vi "image_reg_coke_can.vi"() -> ()   [LabVIEW 2012]
uses:
  Labmembers/Lukas Gemar/Control 1.ctl
  <vilib>/DAQmx/write.llb/DAQmx Write (Digital Bool 1Line 1Point).vi
  <vilib>/Analysis/baseanly.llb/Mean (DBL).vi
  <vilib>/DAQmx/create/channels.llb/DAQmx Create Channel (DO-Digital Output).vi
  <vilib>/DAQmx/miscellaneous.llb/DAQmx Fill In Error Info.vi
  <vilib>/Analysis/NI_AALBase.lvlib
panel:
  in  "Bin (n x n) 2":u16(ring)=1 caption="Cursor Bin" items=["1x1"=1, "2x2"=2, "4x4"=4]
  out "Status":string="Ready"
  in  "Tab Control":enum32{"Page 1", "Page 2", "Page 3"}(tab)
  out "Initialize":u32
  out "Initialize?":bool
  out "Bits per Channel":i32
  out "camera initialization error":errorcluster
  out "Camera ID":string="0"
  out "Model":string="0"
  out "y pixels":i32
  out "x pixels":i32
  out "Elapsed time (sec)":dbl=100.0 min=1.0 max=5000.0 step=1.0
  out "Total time (sec)":dbl=100.0 min=1.0 max=5000.0 step=1.0
  in  "# frames":u32=100
  in  "Acquire movie":bool
  in  "Previous ROI 2":bool
  out "Previous ROI":T1={"x offset"=256, "y offset"=256, "x width"=512, "y width"=512} caption="Previous" {"x offset" min=1 max=512 step=1; "y offset" min=1 max=512 step=1; "x width" min=1 max=512 step=1; "y width" min=1 max=512 step=1}
  in  "Update ROI":bool
  out "ROI":T1={"x offset"=960, "y offset"=912, "x width"=136, "y width"=152} caption="Current" {"x offset" min=1 max=512 step=1; "y offset" min=1 max=512 step=1; "x width" min=1 max=512 step=1; "y width" min=1 max=512 step=1}
  in  "Bin (n x n)":u16(ring)=1 caption="Cursor Bin" items=["1x1"=1, "2x2"=2, "4x4"=4]
  in  "Symmetrical":bool=TRUE
  in  "Define ROI":bool
  in  "ROI selection":u16(ring)=2 items=["Full ROI", "Central quad", "Custom ROI"]
  out "Frames Recorded":i32
  in  "Movie name":string
  in  "Register!":bool
  in  "Image Registration":bool
  in  "Stop Program":bool
  in  "Enter Live Mode":bool
  out "Image":i32[][](graph)
  out "mean":dbl=701.2764784557547
  out "max value":u16=1056
  out "min value":u16=384
  out "Histogram":T2(graph)={"X Values"=[417.6, 484.8, 552.0, 619.2, 686.4, 753.6, 820.8, 888.0, 955.2, 1022.4], "Histogram: h(x)"=[403, 4234, 6440, 8496, 9541, 10568, 10361, 4568, 669, 48]}
  out "Camera Error":errorcluster
  in  "base path":path=path "C:/Peng/Data"
  in  "Exposure (msec)":T3=100.0
  out "Location indicator":u16[][](graph)
  out "max frame rate (Hz)":dbl
  in  "Image Reg Path":path=path "C:/data/Lukas_data/image_reg.bin"
  out "DeviceID":u32
  out "SequID":u32
  in  "DMD_trigger":tag="Dev1/port0/line0" caption="DMD trigger"
  in  "DAQ Error":errorcluster
  in  "Image Reg ctl points":path=path "C:/data/Lukas_data/image_reg.txt"
  in  "Transformation":path=path "C:/data/Lukas_data/transform.txt"
  out "DevFreeErr":i32
  out "SeqFreeErr":i32
  out "ALP_Error":errorcluster
  out "Previous Bin":u16(ring)=2 caption="Cursor Bin" items=["1x1"=1, "2x2"=2, "4x4"=4]
  out "ROI cursor":T1={"x offset"=480, "y offset"=456, "x width"=68, "y width"=76} {"x offset" min=1 max=512 step=1; "y offset" min=1 max=512 step=1; "x width" min=1 max=512 step=1; "y width" min=1 max=512 step=1}
  # "ROI control"
  # "Focus mode settings"
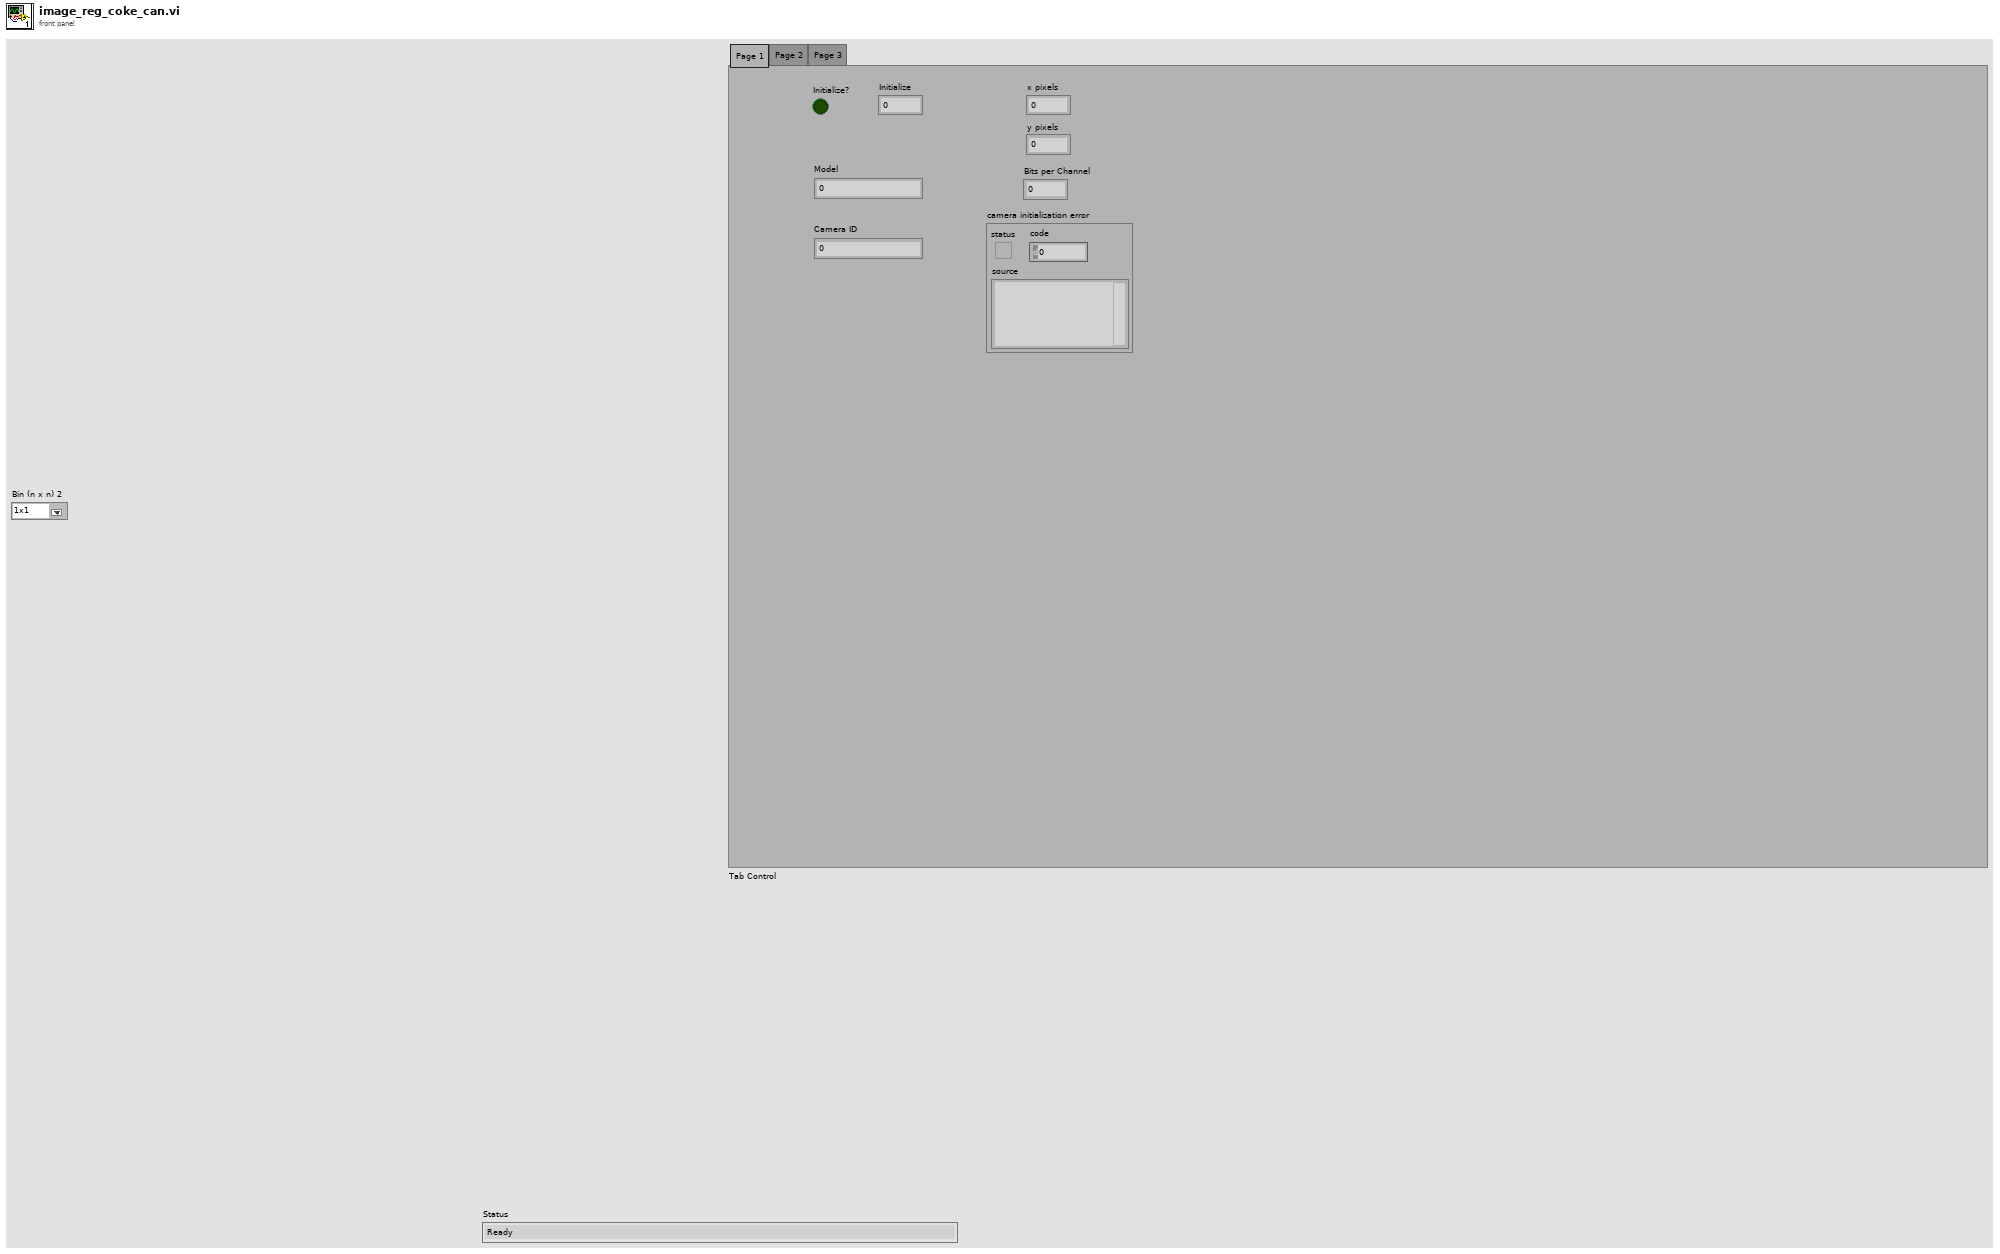
[diagram p1: front panel]
types:
  T1 = cluster{"x offset":i32, "y offset":i32, "x width":i32, "y width":i32}
  T2 = cluster{"X Values":dbl[], "Histogram: h(x)":i32[]}
  T3 = typedef "Control 1.ctl" = dbl
  T4 = cluster{"width":u32, "height":u32, "datatype":u32}
  T5 = enum8{"Enabled", "Disabled", "Disabled and Grayed Out"}
  T6 = cluster{"Horizontal Offset":i32, "Vertical Offset":i32, "Horizontal Width":i32, "Vertical Width":i32}
  T7 = cluster{"Value":i32, "Minimum":i32, "Maximum":i32, "Increment":i32}
  T8 = cluster{"X min":dbl, "Y min":dbl, "X max":dbl, "Y max":dbl}
  T9 = cluster{"Cursor.Cursor X":dbl, "Cursor.Cursor Y":dbl, "Cursor.Cursor X":dbl, "Cursor.Cursor Y":dbl}
  T10 = cluster{"Cursor1. X":dbl, "Cursor1. Y":dbl, "Cursor2. X":dbl, "Cursor2. Y":dbl}
  T11 = cluster{"x offset":dbl, "y offset":dbl, "x width":dbl, "y width":dbl}
  T12 = typedef "LVPointDoubleTypeDef.ctl" = cluster{"Cursor X":dbl, "Cursor Y":dbl}
  T13 = cluster{"XScale.Minimum":dbl, "YScale.Minimum":dbl, "XScale.Maximum":dbl, "YScale.Maximum":dbl}
  T14 = cluster{"Cursor.Cursor Position":T12, "Cursor.Cursor Position":T12}
  T15 = cluster{"Cursor1.Position":T12, "Cursor2.Position":T12}
  T16 = cluster{"Active Cursor":u32, "Active Cursor":u32, dbl, dbl}
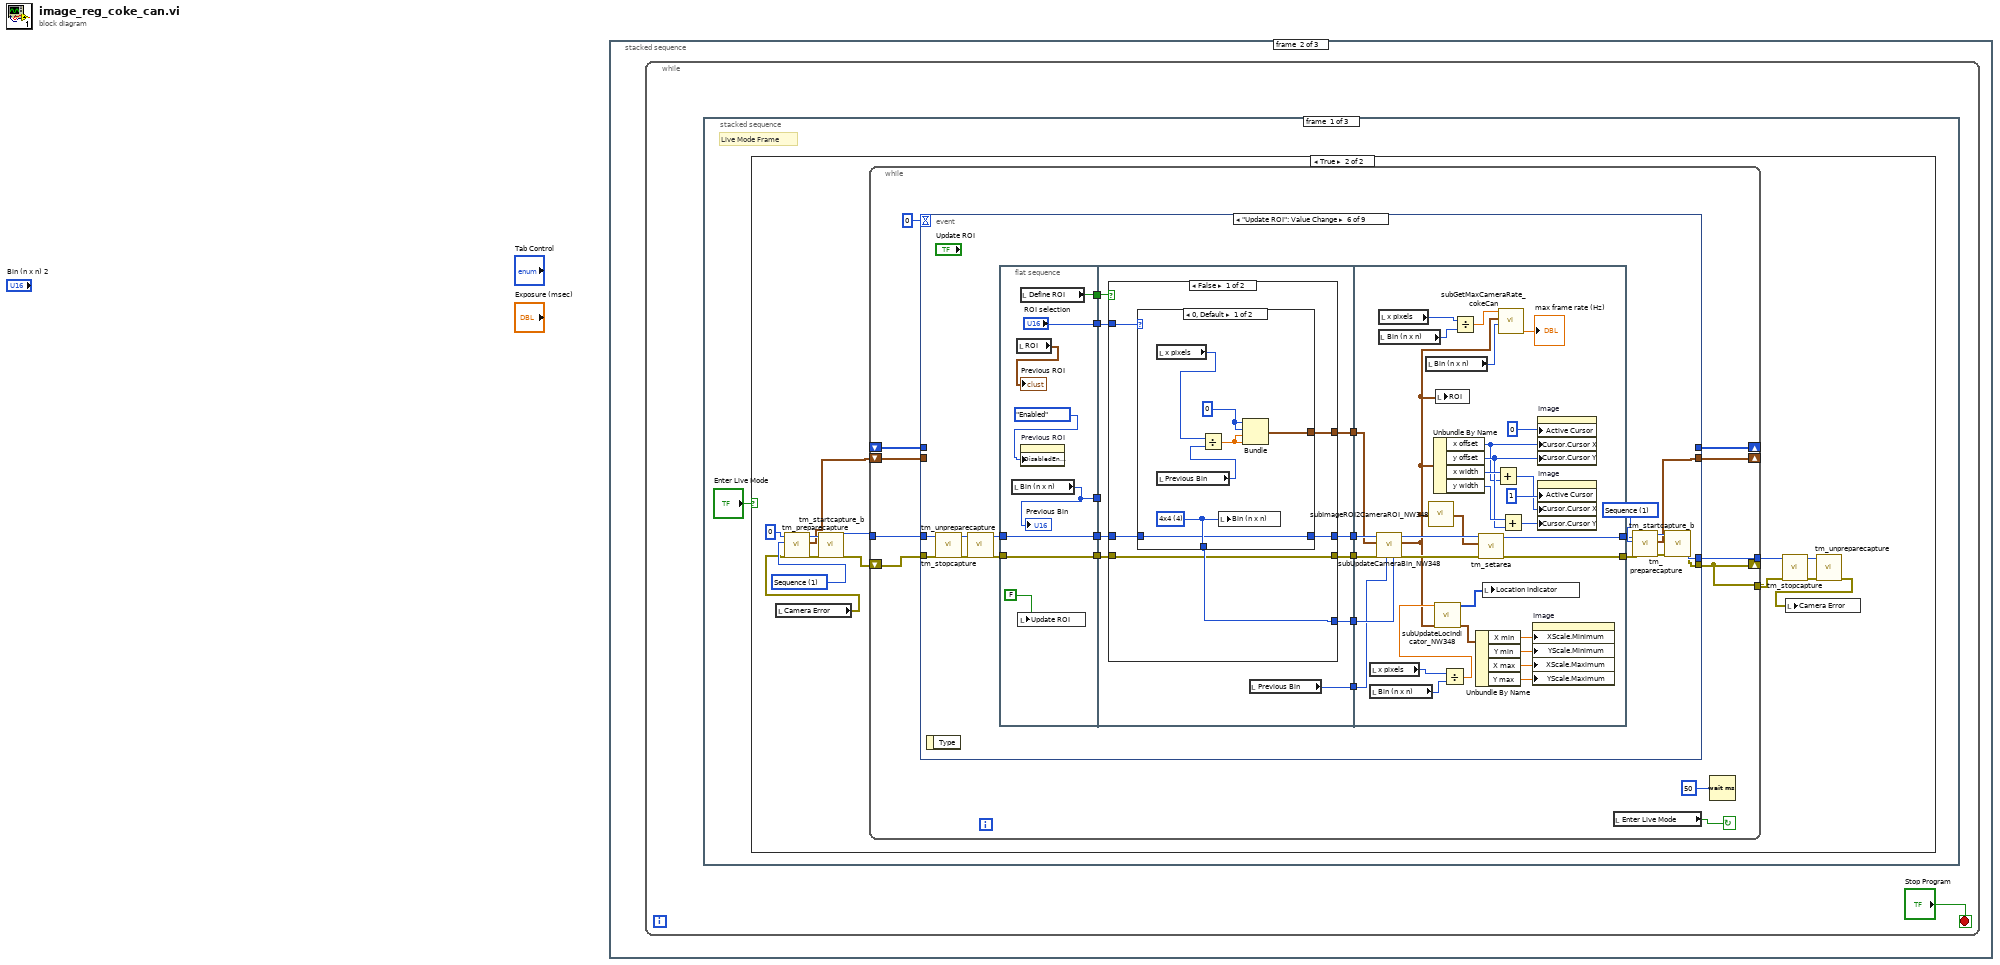
[diagram p0: block diagram]
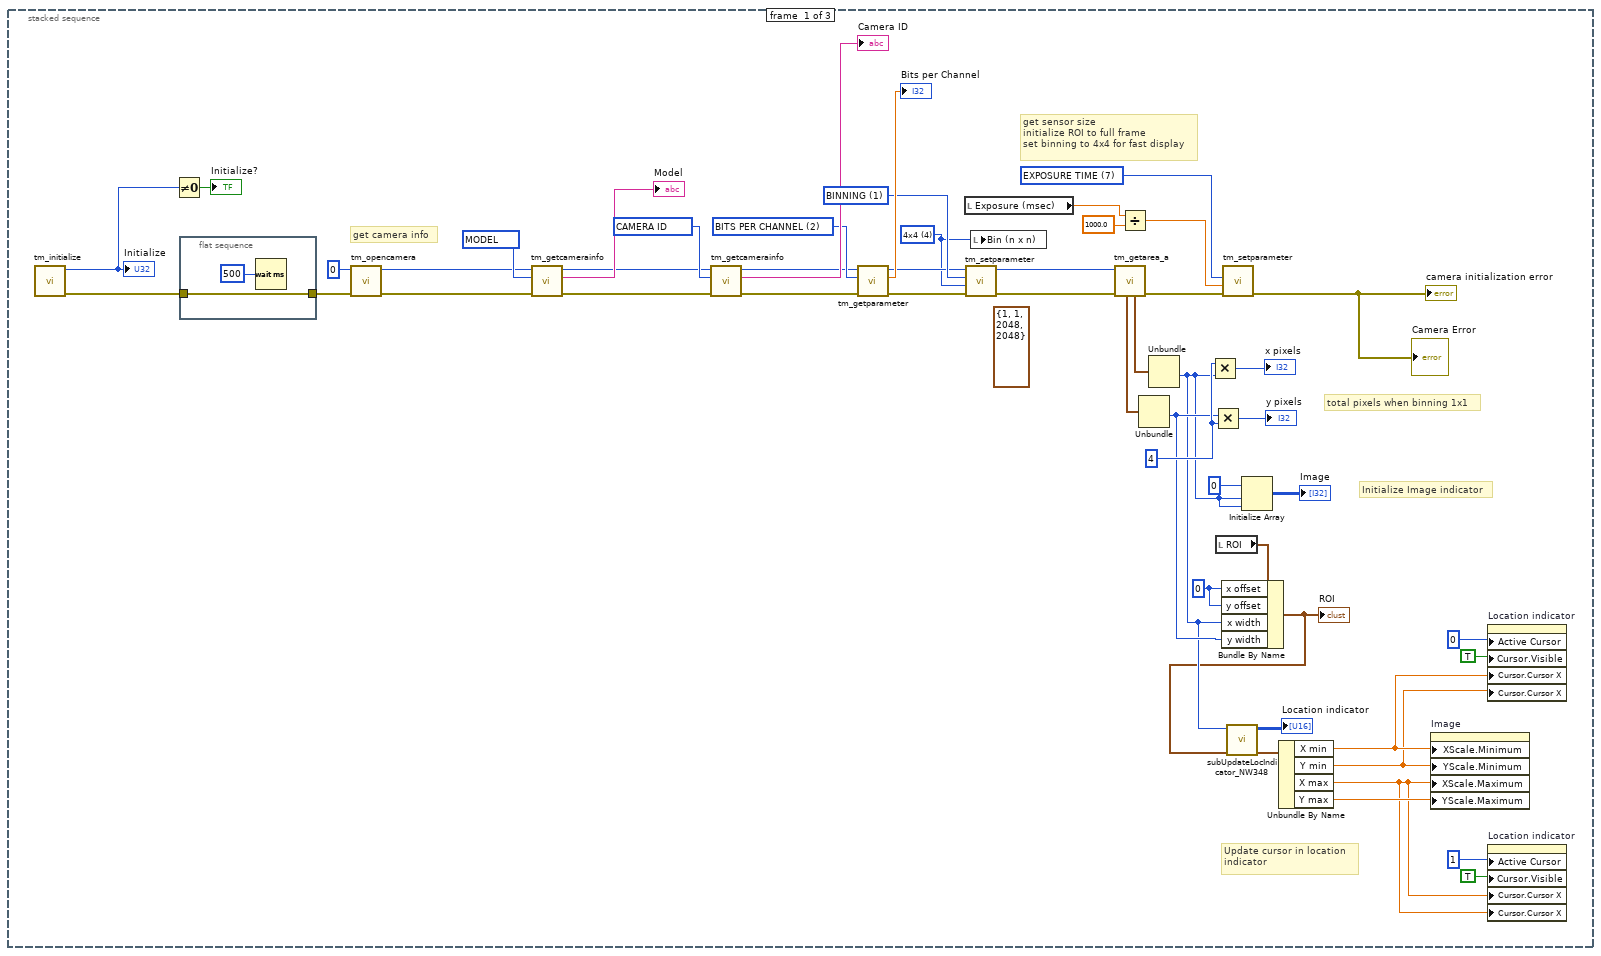
[diagram p2: hidden frame]
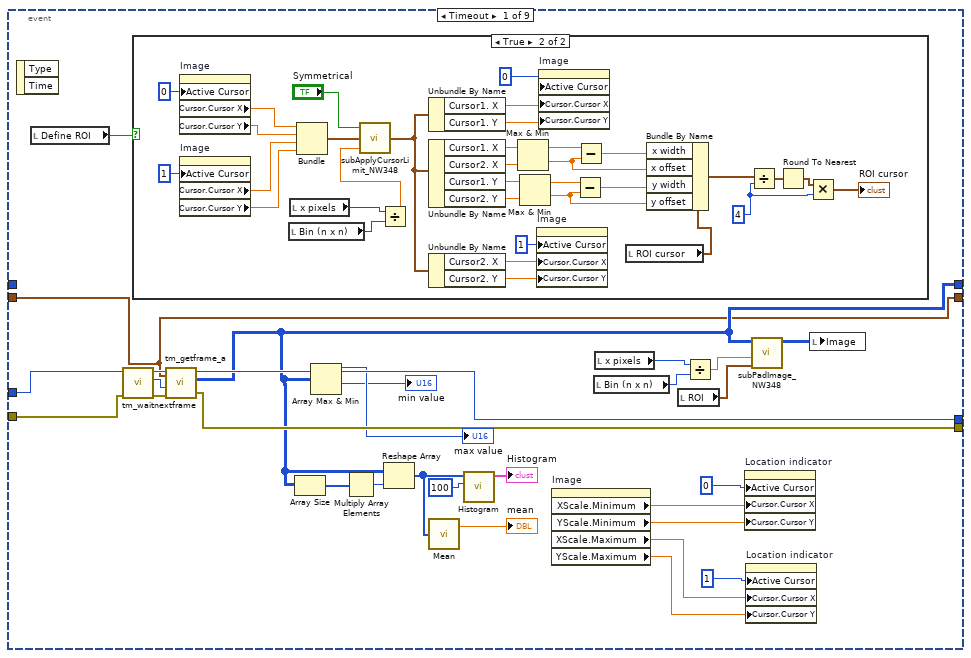
[diagram p4: hidden frame]
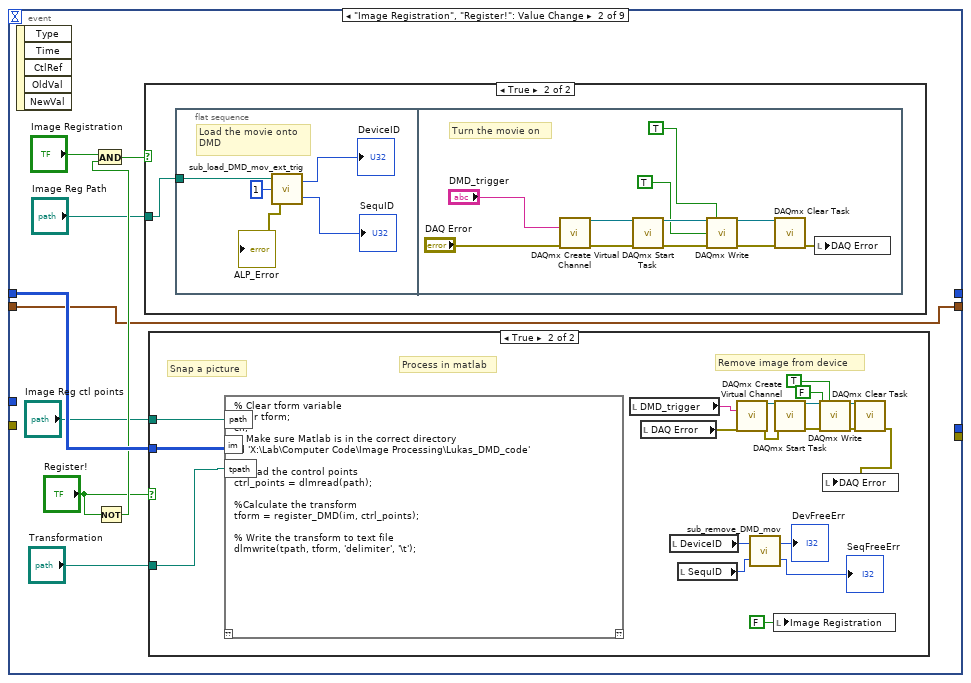
[diagram p6: hidden frame]
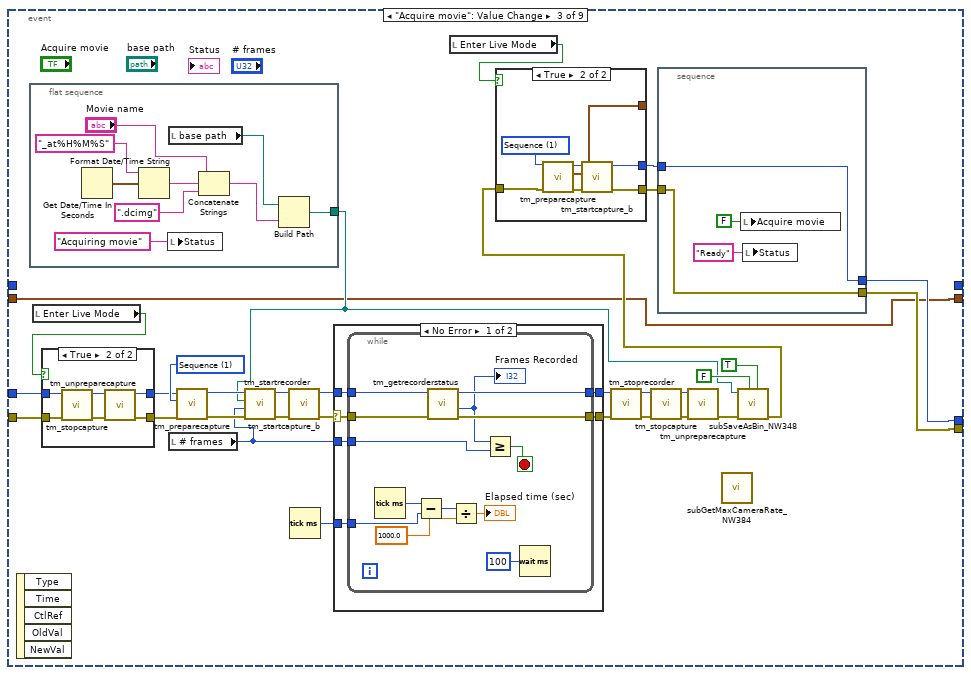
[diagram p9: hidden frame]
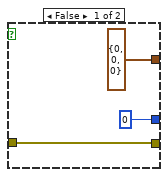
[diagram p10: hidden frame]
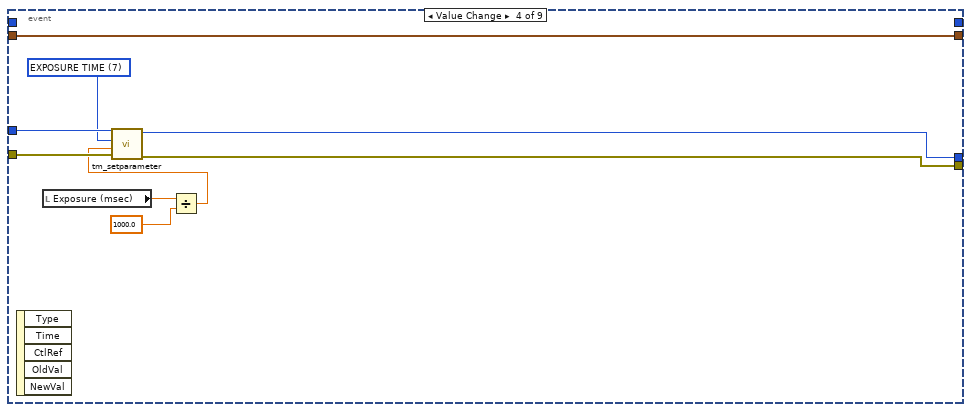
[diagram p13: hidden frame]
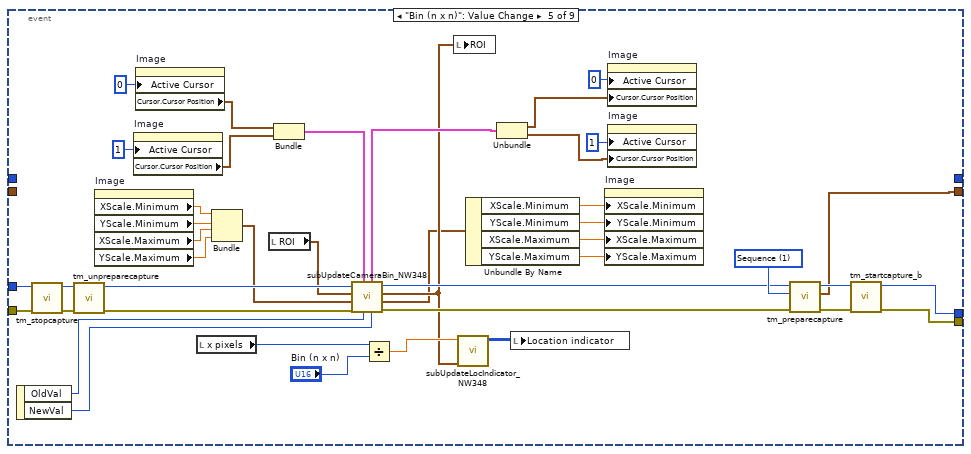
[diagram p14: hidden frame]
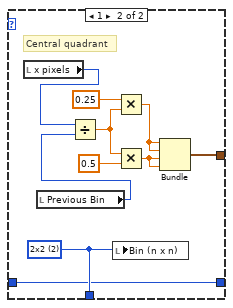
[diagram p15: hidden frame]
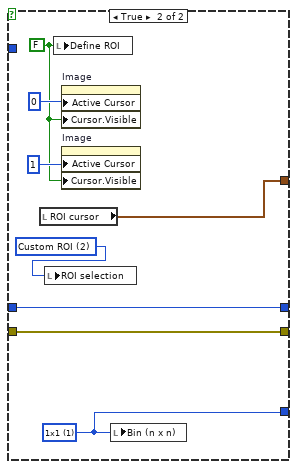
[diagram p16: hidden frame]
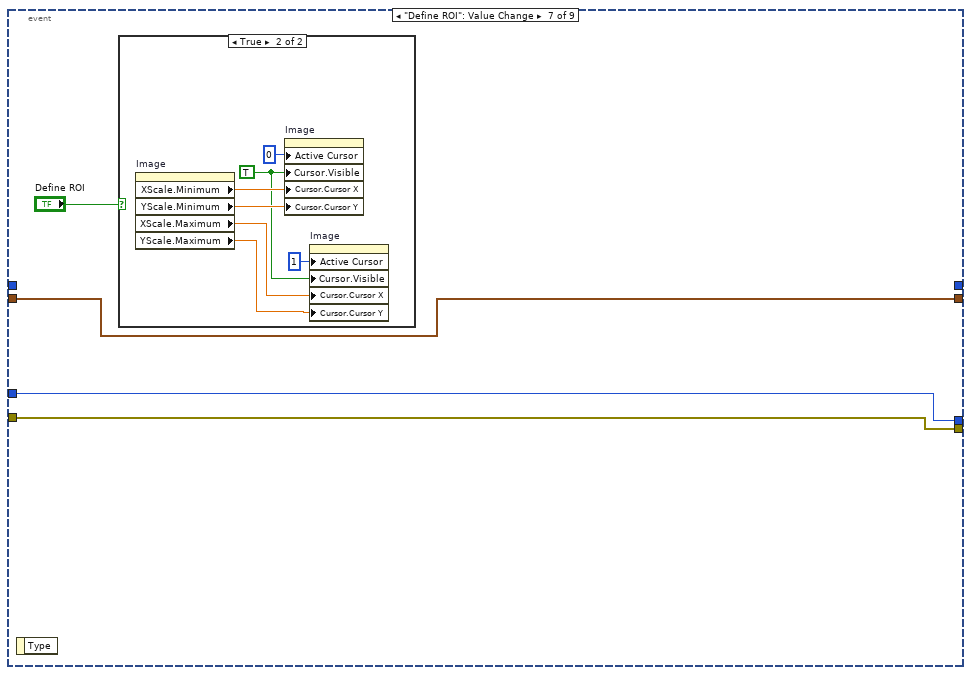
[diagram p17: hidden frame]
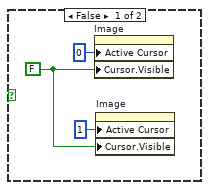
[diagram p18: hidden frame]
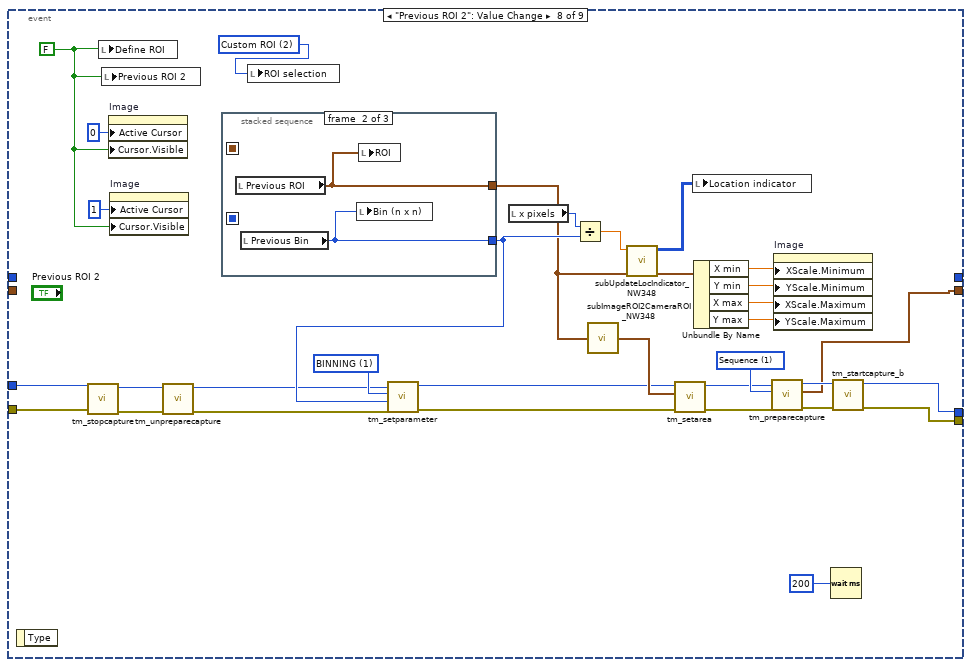
[diagram p19: hidden frame]
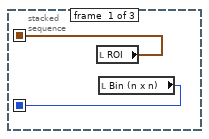
[diagram p20: hidden frame]
diagram:
  n1 = stacked-sequence {
    frame #0 {
      w16 = 0 ("x offset")
      w28 = 4
      (unwired) T6 {"Horizontal Offset"=1, "Vertical Offset"=1, "Horizontal Width"=2048, "Vertical Width"=2048} ("Sub Region")
      w1 = u16 4 items=["1x1"=1, "2x2"=2, "4x4"=4] ("Bin (n x n)")
      w35 = 7 items=["BINNING"=1, "BITS PER CHANNEL"=2, "ACTIVE VIEW INDEX"=3, "CCD MODE"=4, "SENSOR MODE"=5, "READOUT MODE"=6, "EXPOSURE TIME"=7, "CONTRAST GAIN"=8, "CONTRAST OFFSET"=9, "LIGHT MODE"=10, "SENSITIVITY"=11, "WHITE BALANCE"=12, "PHOTON IMAGING MODE"=13, "HIGH DYNAMIC RANGE MODE"=14, "TRIGGER SOURCE"=15, "TRIGGER ACTIVE"=16, "TRIGGER MODE"=17, "TRIGGER POLARITY"=18, "TRIGGER GLOBAL EXPOSURE"=19, "FIRST TRIGGER BEHAVIOR"=20, "TRIGGER TIMES"=21, "OUTPUT TRIGGER POLARITY"=22, "OUTPUT TRIGGER DELAY"=23, "OUTPUT TRIGGER PERIOD"=24, "TEMPERATURE"=25, "TEMPERATURE TARGET"=26, "SENSOR COOLER FAN"=27, "MECHANICAL SHUTTER"=28, "BACK FOCUS POSITION"=29, "FRAMEBUNDLE MODE"=30, "FRAMEBUNDLE NUMBER"=31, "LINEBUNDLE HEIGHT"=32, "TRIGGER CONNECTOR"=33, "IMAGE PIXEL TYPE"=34] ("Parameter")
      w39 = 1 items=["BINNING"=1, "BITS PER CHANNEL"=2, "ACTIVE VIEW INDEX"=3, "CCD MODE"=4, "SENSOR MODE"=5, "READOUT MODE"=6, "EXPOSURE TIME"=7, "CONTRAST GAIN"=8, "CONTRAST OFFSET"=9, "LIGHT MODE"=10, "SENSITIVITY"=11, "WHITE BALANCE"=12, "PHOTON IMAGING MODE"=13, "HIGH DYNAMIC RANGE MODE"=14, "TRIGGER SOURCE"=15, "TRIGGER ACTIVE"=16, "TRIGGER MODE"=17, "TRIGGER POLARITY"=18, "TRIGGER GLOBAL EXPOSURE"=19, "FIRST TRIGGER BEHAVIOR"=20, "TRIGGER TIMES"=21, "OUTPUT TRIGGER POLARITY"=22, "OUTPUT TRIGGER DELAY"=23, "OUTPUT TRIGGER PERIOD"=24, "TEMPERATURE"=25, "TEMPERATURE TARGET"=26, "SENSOR COOLER FAN"=27, "MECHANICAL SHUTTER"=28, "BACK FOCUS POSITION"=29, "FRAMEBUNDLE MODE"=30, "FRAMEBUNDLE NUMBER"=31, "LINEBUNDLE HEIGHT"=32, "TRIGGER CONNECTOR"=33, "IMAGE PIXEL TYPE"=34] ("Parameter")
      w41 = 2 items=["BINNING"=1, "BITS PER CHANNEL"=2, "ACTIVE VIEW INDEX"=3, "CCD MODE"=4, "SENSOR MODE"=5, "READOUT MODE"=6, "EXPOSURE TIME"=7, "CONTRAST GAIN"=8, "CONTRAST OFFSET"=9, "LIGHT MODE"=10, "SENSITIVITY"=11, "WHITE BALANCE"=12, "PHOTON IMAGING MODE"=13, "HIGH DYNAMIC RANGE MODE"=14, "TRIGGER SOURCE"=15, "TRIGGER ACTIVE"=16, "TRIGGER MODE"=17, "TRIGGER POLARITY"=18, "TRIGGER GLOBAL EXPOSURE"=19, "FIRST TRIGGER BEHAVIOR"=20, "TRIGGER TIMES"=21, "OUTPUT TRIGGER POLARITY"=22, "OUTPUT TRIGGER DELAY"=23, "OUTPUT TRIGGER PERIOD"=24, "TEMPERATURE"=25, "TEMPERATURE TARGET"=26, "SENSOR COOLER FAN"=27, "MECHANICAL SHUTTER"=28, "BACK FOCUS POSITION"=29, "FRAMEBUNDLE MODE"=30, "FRAMEBUNDLE NUMBER"=31, "LINEBUNDLE HEIGHT"=32, "TRIGGER CONNECTOR"=33, "IMAGE PIXEL TYPE"=34] ("Parameter")
      w45 = u32 67109122 items=["BUS"=67109121, "CAMERA ID"=67109122, "VENDOR"=67109123, "MODEL"=67109124, "CAMERA VERSION"=67109125, "DRIVER VERSION"=67109126, "MODULE VERSIOIN"=67109127, "DCAMAPI VERSION"=67109128] ("Info ID")
      w44 = u32 67109124 items=["BUS"=67109121, "CAMERA ID"=67109122, "VENDOR"=67109123, "MODEL"=67109124, "CAMERA VERSION"=67109125, "DRIVER VERSION"=67109126, "MODULE VERSIOIN"=67109127, "DCAMAPI VERSION"=67109128] ("Info ID")
      # "Update cursor in location\nindicator"
      # "total pixels when binning 1x1"
      # "Initialize Image indicator"
      # "get sensor size\ninitialize ROI to full frame\nset binning to 4x4 for fast display"
      # "get camera info"
      n2 = call <userlib>:"tm_initialize.vi"() -> ("error out"=w38:errorcluster, "Number Of Cameras"=w49:u32)  [unwired: 10 in]
      "Initialize" <- w49
      n3 = Not Equal To 0?(x=w49) -> (x != 0?=→"Initialize?":bool)
      n4 = flat-sequence {
        tunnel: w38 -> [w52]
        tunnel: [w52] -> w37
        frame #0 {
          n5 = Wait (ms)(milliseconds to wait=u32 500) -> ()  [unwired: 1 out]
        }
      }
      n6 = call <userlib>:"tm_opencamera.vi"("error in (no error)"=w37, "Camera Index"=u32 0 ("milliseconds to wait")) -> ("error out"=w47:errorcluster, "Handle out"=w25:u32)  [unwired: 8 in]
      n7 = call <userlib>:"tm_getcamerainfo.vi"("error in (no error)"=w47, "Info ID"=w44, "Handle in"=w25) -> ("error out"=w43:errorcluster, "String"=→"Model":string, "Handle out"=w24:u32)  [unwired: 6 in]
      n8 = call <userlib>:"tm_getcamerainfo.vi"("error in (no error)"=w43, "Info ID"=w45, "Handle in"=w24) -> ("error out"=w32:errorcluster, "String"=→"Camera ID":string, "Handle out"=w23:u32)  [unwired: 6 in]
      n9 = call <userlib>:"tm_getparameter.vi"("error in (no error)"=w32, "Parameter"=w41, "Handle in"=w23) -> ("error out"=w34:errorcluster, "Value out"=→"Bits per Channel":dbl, "Handle out"=w22:u32)  [unwired: 6 in]
      n10 = local read "Exposure (msec)"() -> (w21:T3)
      n11 = call <userlib>:"tm_setparameter.vi"("error in (no error)"=w34, "Value in"=w1, "Parameter"=w39, "Handle in"=w22) -> ("error out"=w9:errorcluster, "Handle out"=w10:u32)  [unwired: 6 in]
      n12 = local write "Bin (n x n)"(w1) -> ()
      n13 = call <userlib>:"tm_getarea_a.vi"("error in (no error)"=w9, "Handle in"=w10) -> ("error out"=w36:errorcluster, "H Width"=w30:T7, "V Width"=w29:T7)  [unwired: 4 in, 3 out]
      n14 = Divide(x=w21, y=1000.0) -> (x/y=w50:T3)
      n15 = Unbundle(w29) -> ("Maximum"=w17:i32)  [unwired: 3 out]
      n16 = Unbundle(w30) -> ("Maximum"=w15:i32)  [unwired: 3 out]
      n17 = Multiply(x=w28, y=w15) -> (x*y=→"x pixels":i32)
      n18 = Multiply(x=w17, y=w28) -> (x*y=→"y pixels":i32)
      n19 = local read "ROI"() -> (w18:T1)
      n20 = Bundle By Name(cluster=w18, "x offset"=w16, "y offset"=w16, "x width"=w15, "y width"=w17) -> (w14:T1)
      "ROI" <- w14
      n21 = call <userlib>:"tm_setparameter.vi"("error in (no error)"=w36, "Value in"=w50, "Parameter"=w35) -> ("error out"=→"camera initialization error" →"Camera Error":errorcluster)  [unwired: 7 in, 1 out]
      n22 = call "subUpdateLocIndicator_NW348.vi"("ROI"=w14, "pixel range"=w15) -> ("Graph scale"=w13:T8, "Location indicator"=→"Location indicator":u16[][])  [unwired: 8 in]
      n23 = Initialize Array(0, w15, w15) -> (→"Image":i32[][])
      n24 = Unbundle By Name(w13) -> ("X min"=w6:dbl, "Y min"=w5:dbl, "X max"=w2:dbl, "Y max"=w12:dbl)
      n25 = property on="Image" class="IntGraph (strict)"("XScale.Minimum"=w6, "YScale.Minimum"=w5, "XScale.Maximum"=w2, "YScale.Maximum"=w12) -> ()  [unwired: 2 in, 2 out]
      n26 = property on="Location indicator" class="IntGraph (strict)"("Active Cursor"=0 ("x offset"), "Cursor.Visible"=TRUE, "Cursor.Cursor X"=w6, "Cursor.Cursor X"=w5) -> ()  [unwired: 2 in, 2 out]
      n27 = property on="Location indicator" class="IntGraph (strict)"("Active Cursor"=1 ("x offset"), "Cursor.Visible"=TRUE, "Cursor.Cursor X"=w2, "Cursor.Cursor X"=w2) -> ()  [unwired: 2 in, 2 out]
    }
    frame #1 {
      n28 = while {
        stop <- "Stop Program" stop-if-true
        n29 = stacked-sequence {
          frame #0 {
            # "Live Mode Frame"
            n30 = case shown="True" "Enter Live Mode" {
              frame False {
              }
              frame True {
                w68 = 1 items=["Snap", "Sequence"] ("Capture mode")
                n31 = local read "Camera Error"() -> (w57:errorcluster)
                n32 = call <userlib>:"tm_preparecapture.vi"("error in (no error)"=w57, "Capture mode"=w68, "Handle in"=u32 0) -> ("error out"=w66:errorcluster, "Buffer"=w56:T4, "Handle out"=w67:u32)  [unwired: 5 in, 1 out]
                n33 = call <userlib>:"tm_startcapture_b.vi"("error in (no error)"=w66, "Handle in"=w67) -> ("error out"=w64:errorcluster, "Handle out"=w63:u32)  [unwired: 8 in]
                n34 = while {
                  tunnel: [w78] -> w59
                  shift-right: [w75] -> _
                  shift-left: w64 -> [w77]
                  tunnel: w63 -> [w76]
                  tunnel: [w75] -> w60
                  shift-right: [w72] -> _
                  shift-left: _ -> [w71]
                  shift-right: [w70] -> _
                  shift-left: w56 -> [w69]
                  stop <- w79 continue-if-true
                  n35 = event shown="[5] \"Update ROI\": Value Change" {
                    selector: _ -> [_ _ _ _ _ _ _ _ _]
                    dyn-events: _ -> [_ _ _ _ _ _ _ _ _]
                    timeout: 0 -> [_ _ _ _ _ _ _ _ _]
                    tunnel: [w108 _ w191 w277 w289 w335 w429 w450 _] -> w78
                    tunnel: w77 -> [w107 _ w218 w275 w320 w327 w428 w443 _]
                    tunnel: w76 -> [w106 _ w217 w279 w321 w326 w429 w444 _]
                    tunnel: [w105 _ w190 w276 w288 w334 w428 w449 _] -> w75
                    tunnel: [w81 _ _ _ _ _ _ _ _] -> w72
                    tunnel: w71 -> [_ w151 _ _ _ _ _ _ _]
                    tunnel: [w80 w143 w188 w271 w292 w333 w427 w442 w480] -> w70
                    tunnel: w69 -> [w80 w143 w188 w271 _ _ w427 _ w480]
                    event Timeout {
                      n36 = event-data() -> ()  [unwired: 1 in, 2 out]
                      n37 = local read "Define ROI"() -> (w95:bool)
                      n38 = call <userlib>:"tm_waitnextframe.vi"("error in (no error)"=w107, "Handle in"=w106) -> ("error out"=w97:errorcluster, "Frame Index"=w99:i32, "Handle out"=w98:u32)  [unwired: 6 in, 1 out]
                      n39 = case shown="True" w95 {
                        frame False {
                        }
                        frame True {
                          w110 = u32 4 ("Active Cursor")
                          n40 = property on="Image" class="IntGraph (strict)"("Active Cursor"=u32 0) -> ("Cursor.Cursor X"=w138:dbl, "Cursor.Cursor Y"=w137:dbl)  [unwired: 2 in, 2 out]
                          n41 = property on="Image" class="IntGraph (strict)"("Active Cursor"=u32 1) -> ("Cursor.Cursor X"=w140:dbl, "Cursor.Cursor Y"=w139:dbl)  [unwired: 2 in, 2 out]
                          n42 = local read "Bin (n x n)"() -> (w134:u16)
                          n43 = local read "x pixels"() -> (w133:i32)
                          n44 = Bundle("Cursor.Cursor X"=w138, "Cursor.Cursor Y"=w137, "Cursor.Cursor X"=w140, "Cursor.Cursor Y"=w139) -> (w136:T9)  [unwired: 1 in]
                          n45 = Divide(x=w133, y=w134) -> (x/y=w132:dbl)
                          n46 = call "subApplyCursorLimit_NW348.vi"("Cursor limit"=w132, "Cursor input"=w136, "Symmetrical ROI"="Symmetrical") -> ("Cursor output"=w131:T10)  [unwired: 2 in]
                          n47 = Unbundle By Name(w131) -> ("Cursor1. X"=w129:dbl, "Cursor1. Y"=w128:dbl)
                          n48 = Unbundle By Name(w131) -> ("Cursor1. X"=w124:dbl, "Cursor2. X"=w123:dbl, "Cursor1. Y"=w121:dbl, "Cursor2. Y"=w122:dbl)
                          n49 = Unbundle By Name(w131) -> ("Cursor2. X"=w126:dbl, "Cursor2. Y"=w125:dbl)
                          n50 = Max & Min(x=w124, y=w123) -> (max(x,y)=w120:dbl, min(x,y)=w118:dbl)
                          n51 = Max & Min(x=w121, y=w122) -> (max(x,y)=w119:dbl, min(x,y)=w115:dbl)
                          n52 = property on="Image" class="IntGraph (strict)"("Active Cursor"=u32 1, "Cursor.Cursor X"=w126, "Cursor.Cursor Y"=w125) -> ()  [unwired: 2 in, 2 out]
                          n53 = property on="Image" class="IntGraph (strict)"("Active Cursor"=u32 0, "Cursor.Cursor X"=w129, "Cursor.Cursor Y"=w128) -> ()  [unwired: 2 in, 2 out]
                          n54 = Subtract(x=w119, y=w115) -> (x-y=w116:dbl)
                          n55 = Subtract(x=w120, y=w118) -> (x-y=w117:dbl)
                          n56 = local read "ROI cursor"() -> (w114:T1)
                          n57 = Bundle By Name(cluster=w114, "x width"=w117, "x offset"=w118, "y width"=w116, "y offset"=w115) -> (w113:T1)
                          n58 = Divide(x=w113, y=w110) -> (x/y=w112:T11)
                          n59 = Round To Nearest(number=w112) -> (nearest integer value=w111:T11)
                          n60 = Multiply(x=w111, y=w110) -> (x*y=→"ROI cursor":T11)
                        }
                      }
                      n61 = call <userlib>:"tm_getframe_a.vi"("error in (no error)"=w97, "Frame Index"=w99, "Buffer"=w80, "Handle in"=w98) -> ("error out"=w105:errorcluster, "Data 16"=w81:u16[][], "Handle out"=w108:u32)  [unwired: 4 in, 1 out]
                      n62 = Array Size(array=w81) -> (size(s)=w82:i32[])
                      n63 = Array Max & Min(array=w81) -> (max value=→"max value":u16, min value=→"min value":u16)  [unwired: 2 out]
                      n64 = Multiply Array Elements(1:w82) -> (0:w83:i32)
                      n65 = Reshape Array(w81, w83) -> (w104:u16[])
                      n66 = call-poly <vilib>:"Mean.vi"("X"=w104) -> ("mean"=→"mean":dbl)  [unwired: 1 out]
                      n67 = call <vilib>:"Histogram.vi"("intervals"=100, "X"=w104) -> ("Histogram Graph"=→"Histogram":T2)  [unwired: 6 in, 3 out]
                      n68 = property on="Image" class="IntGraph (strict)"() -> ("XScale.Minimum"=w92:dbl, "YScale.Minimum"=w91:dbl, "XScale.Maximum"=w90:dbl, "YScale.Maximum"=w89:dbl)  [unwired: 2 in, 2 out]
                      n69 = local read "Bin (n x n)"() -> (w86:u16)
                      n70 = local read "x pixels"() -> (w87:i32)
                      n71 = local read "ROI"() -> (w84:T1)
                      n72 = Divide(x=w87, y=w86) -> (x/y=w85:dbl)
                      n73 = property on="Location indicator" class="IntGraph (strict)"("Active Cursor"=0 ("x offset"), "Cursor.Cursor X"=w92, "Cursor.Cursor Y"=w91) -> ()  [unwired: 2 in, 2 out]
                      n74 = property on="Location indicator" class="IntGraph (strict)"("Active Cursor"=1 ("x offset"), "Cursor.Cursor X"=w90, "Cursor.Cursor Y"=w89) -> ()  [unwired: 2 in, 2 out]
                      n75 = call "subPadImage_NW348.vi"("ROI"=w84, "Full size"=w85, "Image in"=w81) -> ("Image out"=w88:u16[][])  [unwired: 7 in, 1 out]
                      n76 = local write "Image"(w88) -> ()
                    }
                    event "Image Registration", "Register!": Value Change {
                      n77 = event-data() -> ()  [unwired: 1 in, 5 out]
                      n78 = Not(x="Register!") -> (.not. x?=w149:bool)
                      n79 = And(x="Image Registration", y=w149) -> (x .and. y?=w148:bool)
                      n80 = case shown="True" w148 {
                        tunnel: "Image Reg Path" -> [_ w171]
                        frame False {
                        }
                        frame True {
                          n81 = flat-sequence {
                            tunnel: w171 -> [w176]
                            frame #0 {
                              # "Load the movie onto\nDMD"
                              n82 = call "sub_load_DMD_mov_ext_trig.vi"("SequenceRepeats"=1, "binary mov path"=w176) -> ("SequID"=→"SequID":u32, "DeviceID"=→"DeviceID":u32, "DevInq1"=→"ALP_Error":errorcluster)
                            }
                            frame #1 {
                              # "Turn the movie on"
                              n83 = call-poly <vilib>:"DAQmx Create Virtual Channel.vi"("lines"="DMD_trigger", "error in"="DAQ Error") -> ("task out"=w182:refnum<k21>, "error out"=w183:errorcluster)  [unwired: 3 in, 9 out]
                              n84 = call <vilib>:"DAQmx Start Task.vi"("task/channels in"=w182, "error in"=w183) -> ("task out"=w184:refnum<k21>, "error out"=w187:errorcluster)  [unwired: 12 out]
                              n85 = call-poly <vilib>:"DAQmx Write.vi"("task/channels in"=w184, "auto start"=TRUE, "data"=TRUE, "error in"=w187) -> ("task out"=w185:refnum<k21>, "error out"=w186:errorcluster)  [unwired: 9 in, 1 out]
                              n86 = call <vilib>:"DAQmx Clear Task.vi"("task in"=w185, "error in"=w186) -> ("error out"=w177:errorcluster)  [unwired: 13 out]
                              n87 = local write "DAQ Error"(w177) -> ()
                            }
                          }
                        }
                      }
                      n88 = case shown="True" "Register!" {
                        tunnel: w151 -> [_ w170]
                        tunnel: "Image Reg ctl points" -> [_ w169]
                        tunnel: "Transformation" -> [_ w168]
                        frame False {
                        }
                        frame True {
                          # "Remove image from device"
                          # "Process in matlab"
                          # "Snap a picture"
                          n89 = script code="% Clear tform variable\nclear tform;\nclf;  \n% Make sure Matlab is in the correct directory\ncd 'X:\\Lab\\Computer Code\\Image Processing\\Lukas_DMD_code'\n\n% Load the control points\nctrl_points = dlmread(path); \n\n%Calculate the transform\ntform = register_DMD(im, ctrl_points); \n\n% Write the transform to text file\ndlmwrite(tpath, tform, 'delimiter', '\\t');"("path"=w169, "im"=w170, "tpath"=w168) -> ()  [unwired: 1 in, 1 out]
                          n90 = local read "DMD_trigger"() -> (w166:tag)
                          n91 = local read "DAQ Error"() -> (w167:errorcluster)
                          n92 = local read "DeviceID"() -> (w156:u32)
                          n93 = local read "SequID"() -> (w155:u32)
                          n94 = call-poly <vilib>:"DAQmx Create Virtual Channel.vi"("lines"=w166, "error in"=w167) -> ("task out"=w165:refnum<k21>, "error out"=w164:errorcluster)  [unwired: 3 in, 9 out]
                          n95 = call "sub_remove_DMD_mov.vi"("SequenceId"=w155, "DeviceId"=w156) -> ("SeqFreeErr"=→"SeqFreeErr":i32, "DevFreeErr"=→"DevFreeErr":i32)
                          n96 = local write "Image Registration"(FALSE ("Image Registration")) -> ()
                          n97 = call <vilib>:"DAQmx Start Task.vi"("task/channels in"=w165, "error in"=w164) -> ("task out"=w163:refnum<k21>, "error out"=w162:errorcluster)  [unwired: 12 out]
                          n98 = call-poly <vilib>:"DAQmx Write.vi"("task/channels in"=w163, "auto start"=TRUE, "data"=FALSE, "error in"=w162) -> ("task out"=w160:refnum<k21>, "error out"=w159:errorcluster)  [unwired: 9 in, 1 out]
                          n99 = call <vilib>:"DAQmx Clear Task.vi"("task in"=w160, "error in"=w159) -> ("error out"=w158:errorcluster)  [unwired: 13 out]
                          n100 = local write "DAQ Error"(w158) -> ()
                        }
                      }
                    }
                    event "Acquire movie": Value Change {
                      w211 = 1 items=["Snap", "Sequence"] ("Capture mode")
                      n101 = event-data() -> ()  [unwired: 1 in, 5 out]
                      n102 = flat-sequence {
                        tunnel: [w270] -> w196
                        frame #0 {
                          n103 = Get Date/Time In Seconds() -> (seconds since 1Jan1904=w264:timestamp)
                          n104 = Format Date/Time String(time format string (%c)="_at%H%M%S", seconds (now)=w264) -> (date/time string=w263:string)  [unwired: 1 in]
                          n105 = local write "Status"("Acquiring movie" ("Status")) -> ()
                          n106 = local read "base path"() -> (w268:path)
                          n107 = Concatenate Strings("Movie name", w263, ".dcimg" ("string")) -> (w269:string)
                          n108 = Build Path(base path=w268, name or relative path=w269) -> (appended path=w270:path)
                        }
                      }
                      n109 = local read "Enter Live Mode"() -> (w216:bool)
                      n110 = case shown="True" w216 {
                        tunnel: [w255 w259] -> w209
                        tunnel: w218 -> [w255 w258]
                        tunnel: w217 -> [w254 w257]
                        tunnel: [w254 w256] -> w210
                        frame False {
                        }
                        frame True {
                          n111 = call <userlib>:"tm_stopcapture.vi"("error in (no error)"=w258, "Handle in"=w257) -> ("error out"=w260:errorcluster, "Handle out"=w261:u32)  [unwired: 8 in]
                          n112 = call <userlib>:"tm_unpreparecapture.vi"("error in (no error)"=w260, "Handle in"=w261) -> ("error out"=w259:errorcluster, "Handle out"=w256:u32)  [unwired: 8 in]
                        }
                      }
                      n113 = local read "# frames"() -> (w189:u32)
                      n114 = call <userlib>:"tm_preparecapture.vi"("error in (no error)"=w209, "Capture mode"=w211, "Handle in"=w210) -> ("error out"=w212:errorcluster, "Handle out"=w213:u32)  [unwired: 5 in, 2 out]
                      n115 = call <userlib>:"tm_startrecorder.vi"("error in (no error)"=w212, "frames"=w189, "File"=w196, "Handle in"=w213) -> ("error out"=w214:errorcluster, "Handle out"=w215:u32)  [unwired: 6 in]
                      n116 = call <userlib>:"tm_startcapture_b.vi"("error in (no error)"=w214, "Handle in"=w215) -> ("error out"=w208:errorcluster, "Handle out"=w207:u32)  [unwired: 8 in]
                      n117 = Tick Count (ms)() -> (millisecond timer value=w197:u32)
                      n118 = case shown="No Error" w208 {
                        selector: w208 -> [w238 w253]
                        tunnel: [w236 w252] -> w201
                        tunnel: [w237 w253] -> w202
                        tunnel: w207 -> [w235 w252]
                        tunnel: w197 -> [w234 _]
                        tunnel: w189 -> [w233 _]
                        frame No Error {
                          n119 = while {
                            tunnel: w238 -> [w250]
                            tunnel: [w249] -> w237
                            tunnel: [w251] -> w236
                            tunnel: w235 -> [w243]
                            tunnel: w234 -> [w240]
                            tunnel: w233 -> [w239]
                            stop <- w248 stop-if-true
                            n120 = Tick Count (ms)() -> (millisecond timer value=w245:u32)
                            n121 = Subtract(x=w245, y=w240) -> (x-y=w244:u32)
                            n122 = call <userlib>:"tm_getrecorderstatus.vi"("error in (no error)"=w250, "Handle"=w243) -> ("error out"=w249:errorcluster, "Count"=w242:i32, "Handle"=w251:u32)  [unwired: 6 in, 1 out]
                            "Frames Recorded" <- w242
                            n123 = Divide(x=w244, y=1000.0) -> (x/y=→"Elapsed time (sec)":dbl)
                            n124 = Greater Or Equal?(x=w242, y=w239) -> (x >= y?=w248:bool)
                            n125 = Wait (ms)(milliseconds to wait=u32 100) -> ()  [unwired: 1 out]
                          }
                        }
                        frame Error {
                        }
                      }
                      n126 = local read "Enter Live Mode"() -> (w194:bool)
                      n127 = call <userlib>:"tm_stoprecorder.vi"("error in (no error)"=w202, "Handle in"=w201) -> ("error out"=w206:errorcluster, "Handle out"=w205:u32)  [unwired: 8 in]
                      n128 = call <userlib>:"tm_stopcapture.vi"("error in (no error)"=w206, "Handle in"=w205) -> ("error out"=w203:errorcluster, "Handle out"=w204:u32)  [unwired: 8 in]
                      n129 = call <userlib>:"tm_unpreparecapture.vi"("error in (no error)"=w203, "Handle in"=w204) -> ("error out"=w200:errorcluster)  [unwired: 8 in, 1 out]
                      n130 = call "subGetMaxCameraRate_NW384.vi"() -> ()  [unwired: 10 in, 2 out]
                      n131 = call "subSaveAsBin_NW348.vi"("Delete .dcimg?"=TRUE, "Save Text file?"=FALSE, "Error in"=w200, ".dcimg file name"=w196) -> ("Error out"=w195:errorcluster)  [unwired: 7 in]
                      n132 = case shown="True" w194 {
                        tunnel: [w223 w229] -> w192
                        tunnel: [u32 0 ("Handle out") w228] -> w193
                        tunnel: [T4 {"width"=0, "height"=0, "datatype"=0} ("Buffer") w227] -> _
                        tunnel: w195 -> [w223 w226]
                        frame False {
                        }
                        frame True {
                          w230 = 1 items=["Snap", "Sequence"] ("Capture mode")
                          n133 = call <userlib>:"tm_preparecapture.vi"("error in (no error)"=w226, "Capture mode"=w230) -> ("error out"=w232:errorcluster, "Buffer"=w227:T4, "Handle out"=w231:u32)  [unwired: 6 in, 1 out]
                          n134 = call <userlib>:"tm_startcapture_b.vi"("error in (no error)"=w232, "Handle in"=w231) -> ("error out"=w229:errorcluster, "Handle out"=w228:u32)  [unwired: 8 in]
                        }
                      }
                      n135 = stacked-sequence {
                        tunnel: [w222] -> w191
                        tunnel: w193 -> [w222]
                        tunnel: w192 -> [w221]
                        tunnel: [w221] -> w190
                        frame #0 {
                          n136 = local write "Acquire movie"(FALSE ("Acquire movie")) -> ()
                          n137 = local write "Status"("Ready" ("Status")) -> ()
                        }
                      }
                    }
                    event Value Change {
                      w278 = 7 items=["BINNING"=1, "BITS PER CHANNEL"=2, "ACTIVE VIEW INDEX"=3, "CCD MODE"=4, "SENSOR MODE"=5, "READOUT MODE"=6, "EXPOSURE TIME"=7, "CONTRAST GAIN"=8, "CONTRAST OFFSET"=9, "LIGHT MODE"=10, "SENSITIVITY"=11, "WHITE BALANCE"=12, "PHOTON IMAGING MODE"=13, "HIGH DYNAMIC RANGE MODE"=14, "TRIGGER SOURCE"=15, "TRIGGER ACTIVE"=16, "TRIGGER MODE"=17, "TRIGGER POLARITY"=18, "TRIGGER GLOBAL EXPOSURE"=19, "FIRST TRIGGER BEHAVIOR"=20, "TRIGGER TIMES"=21, "OUTPUT TRIGGER POLARITY"=22, "OUTPUT TRIGGER DELAY"=23, "OUTPUT TRIGGER PERIOD"=24, "TEMPERATURE"=25, "TEMPERATURE TARGET"=26, "SENSOR COOLER FAN"=27, "MECHANICAL SHUTTER"=28, "BACK FOCUS POSITION"=29, "FRAMEBUNDLE MODE"=30, "FRAMEBUNDLE NUMBER"=31, "LINEBUNDLE HEIGHT"=32, "TRIGGER CONNECTOR"=33, "IMAGE PIXEL TYPE"=34] ("Parameter")
                      n138 = event-data() -> ()  [unwired: 1 in, 5 out]
                      n139 = local read "Exposure (msec)"() -> (w274:T3)
                      n140 = Divide(x=w274, y=1000.0) -> (x/y=w273:T3)
                      n141 = call <userlib>:"tm_setparameter.vi"("error in (no error)"=w275, "Value in"=w273, "Parameter"=w278, "Handle in"=w279) -> ("error out"=w276:errorcluster, "Handle out"=w277:u32)  [unwired: 6 in]
                    }
                    event "Bin (n x n)": Value Change {
                      w295 = 1 items=["Snap", "Sequence"] ("Capture mode")
                      n142 = event-data() -> ("OldVal"=w283:u16, "NewVal"=w282:u16)  [unwired: 1 in]
                      n143 = call <userlib>:"tm_stopcapture.vi"("error in (no error)"=w320, "Handle in"=w321) -> ("error out"=w318:errorcluster, "Handle out"=w319:u32)  [unwired: 8 in]
                      n144 = call <userlib>:"tm_unpreparecapture.vi"("error in (no error)"=w318, "Handle in"=w319) -> ("error out"=w316:errorcluster, "Handle out"=w317:u32)  [unwired: 8 in]
                      n145 = property on="Image" class="IntGraph (strict)"() -> ("XScale.Minimum"=w313:dbl, "YScale.Minimum"=w314:dbl, "XScale.Maximum"=w312:dbl, "YScale.Maximum"=w311:dbl)  [unwired: 2 in, 2 out]
                      n146 = property on="Image" class="IntGraph (strict)"("Active Cursor"=u32 1) -> ("Cursor.Cursor Position"=w306:T12)  [unwired: 2 in, 2 out]
                      n147 = property on="Image" class="IntGraph (strict)"("Active Cursor"=u32 0) -> ("Cursor.Cursor Position"=w307:T12)  [unwired: 2 in, 2 out]
                      n148 = local read "x pixels"() -> (w286:i32)
                      n149 = Bundle("XScale.Minimum"=w313, "YScale.Minimum"=w314, "XScale.Maximum"=w312, "YScale.Maximum"=w311) -> (w310:T13)  [unwired: 1 in]
                      n150 = local read "ROI"() -> (w315:T1)
                      n151 = Bundle("Cursor.Cursor Position"=w307, "Cursor.Cursor Position"=w306) -> (w305:T14)  [unwired: 1 in]
                      n152 = call "subUpdateCameraBin_NW348.vi"("Bin (n x n)"=w282, "Previous bin"=w283, "Cursor in"=w305, "Error in (no error)"=w316, "Graph scale in"=w310, "ROI in"=w315, "Handle in"=w317) -> ("Error out"=w290:errorcluster, "Graph scale out"=w280:T13, "ROI out"=w281:T1, "Handle out"=w291:u32, "Cursor out"=w302:T15)
                      n153 = Divide(x=w286, y="Bin (n x n)") -> (x/y=w284:dbl)
                      n154 = local write "ROI"(w281) -> ()
                      n155 = call "subUpdateLocIndicator_NW348.vi"("ROI"=w281, "pixel range"=w284) -> ("Location indicator"=w285:u16[][])  [unwired: 8 in, 1 out]
                      n156 = Unbundle By Name(w280) -> ("XScale.Minimum"=w299:dbl, "YScale.Minimum"=w298:dbl, "XScale.Maximum"=w297:dbl, "YScale.Maximum"=w296:dbl)
                      n157 = Unbundle(w302) -> ("Cursor1.Position"=w301:T12, "Cursor2.Position"=w300:T12)
                      n158 = local write "Location indicator"(w285) -> ()
                      n159 = property on="Image" class="IntGraph (strict)"("XScale.Minimum"=w299, "YScale.Minimum"=w298, "XScale.Maximum"=w297, "YScale.Maximum"=w296) -> ()  [unwired: 2 in, 2 out]
                      n160 = property on="Image" class="IntGraph (strict)"("Active Cursor"=u32 0, "Cursor.Cursor Position"=w301) -> ()  [unwired: 2 in, 2 out]
                      n161 = property on="Image" class="IntGraph (strict)"("Active Cursor"=u32 1, "Cursor.Cursor Position"=w300) -> ()  [unwired: 2 in, 2 out]
                      n162 = call <userlib>:"tm_preparecapture.vi"("error in (no error)"=w290, "Capture mode"=w295, "Handle in"=w291) -> ("error out"=w293:errorcluster, "Buffer"=w292:T4, "Handle out"=w294:u32)  [unwired: 5 in, 1 out]
                      n163 = call <userlib>:"tm_startcapture_b.vi"("error in (no error)"=w293, "Handle in"=w294) -> ("error out"=w288:errorcluster, "Handle out"=w289:u32)  [unwired: 8 in]
                    }
                    event "Update ROI": Value Change {
                      w338 = 1 items=["Snap", "Sequence"] ("Capture mode")
                      n164 = event-data() -> ()  [unwired: 1 in, 1 out]
                      n165 = call <userlib>:"tm_stopcapture.vi"("error in (no error)"=w327, "Handle in"=w326) -> ("error out"=w325:errorcluster, "Handle out"=w324:u32)  [unwired: 8 in]
                      n166 = call <userlib>:"tm_unpreparecapture.vi"("error in (no error)"=w325, "Handle in"=w324) -> ("error out"=w323:errorcluster, "Handle out"=w322:u32)  [unwired: 8 in]
                      n167 = flat-sequence {
                        tunnel: [w351] -> w345
                        tunnel: [w350] -> w344
                        tunnel: [w349] -> w343
                        tunnel: w322 -> [w349]
                        tunnel: w323 -> [w348]
                        tunnel: [w348] -> w341
                        tunnel: ["ROI selection"] -> w328
                        tunnel: w345 -> [_]
                        tunnel: w344 -> [w362]
                        tunnel: w343 -> [w361]
                        tunnel: [w360] -> w342
                        tunnel: w341 -> [w359]
                        tunnel: [w358] -> w340
                        tunnel: [w357] -> w339
                        tunnel: [w356] -> w330
                        tunnel: [w355] -> w329
                        tunnel: w328 -> [w354]
                        tunnel: w342 -> [w425]
                        tunnel: w340 -> [w426]
                        tunnel: w339 -> [w424]
                        tunnel: [w420] -> w332
                        tunnel: [w419] -> w331
                        tunnel: w330 -> [w401]
                        tunnel: w329 -> [w400]
                        frame #0 {
                          n168 = local read "Bin (n x n)"() -> (w351:u16)
                          "Previous Bin" <- w351
                          n169 = local read "ROI"() -> (→"Previous ROI":T1)
                          n170 = local write "Update ROI"(FALSE ("Update ROI")) -> ()
                          n171 = local read "Define ROI"() -> (w350:bool)
                          n172 = property on="Previous ROI" class="Clust (strict)"("DisabledEnum"=T5."Enabled" ("Disabled")) -> ()  [unwired: 2 in, 2 out]
                        }
                        frame #1 {
                          n173 = case shown="False" w362 {
                            tunnel: [w363 w389] -> w360
                            tunnel: w361 -> [w364 w389]
                            tunnel: w359 -> [w365 w388]
                            tunnel: [w365 w388] -> w358
                            tunnel: [w368 w387] -> w356
                            tunnel: [w367 w386] -> w357
                            tunnel: w354 -> [w366 _]
                            frame False {
                              n174 = case shown="0, Default" w366 {
                                tunnel: [w371 w380] -> w368
                                tunnel: [w370 w379] -> w367
                                tunnel: w364 -> [w369 w376]
                                tunnel: [w369 w376] -> w363
                                frame 0, Default {
                                w371 = u16 4 items=["1x1"=1, "2x2"=2, "4x4"=4] ("Bin (n x n)")
                                w374 = u32 0 ("Active Cursor")
                                n175 = local read "x pixels"() -> (w373:i32)
                                n176 = local read "Previous Bin"() -> (w372:u16)
                                n177 = Divide(x=w373, y=w372) -> (x/y=w375:dbl)
                                n178 = local write "Bin (n x n)"(w371) -> ()
                                n179 = Bundle("Active Cursor"=w374, "Active Cursor"=w374, w375, w375) -> (w370:T16)  [unwired: 1 in]
                                }
                                frame 1 {
                                w380 = u16 2 items=["1x1"=1, "2x2"=2, "4x4"=4] ("Bin (n x n)")
                                # "Central quadrant"
                                n180 = local read "x pixels"() -> (w377:i32)
                                n181 = local read "Previous Bin"() -> (w378:u16)
                                n182 = Divide(x=w377, y=w378) -> (x/y=w381:dbl)
                                n183 = local write "Bin (n x n)"(w380) -> ()
                                n184 = Multiply(x=0.25, y=w381) -> (x*y=w384:dbl)
                                n185 = Multiply(x=w381, y=0.5) -> (x*y=w382:dbl)
                                n186 = Bundle(w384, w384, w382, w382) -> (w379:cluster{dbl, dbl, dbl, dbl})  [unwired: 1 in]
                                }
                              }
                            }
                            frame True {
                              w387 = u16 1 items=["1x1"=1, "2x2"=2, "4x4"=4] ("Bin (n x n)")
                              w390 = u16 2 items=["Full ROI", "Central quad", "Custom ROI"] ("ROI selection")
                              w391 = FALSE ("Define ROI")
                              n187 = local read "ROI cursor"() -> (w386:T1)
                              n188 = local write "ROI selection"(w390) -> ()
                              n189 = local write "Define ROI"(w391) -> ()
                              n190 = property on="Image" class="IntGraph (strict)"("Active Cursor"=u32 0, "Cursor.Visible"=w391) -> ()  [unwired: 2 in, 2 out]
                              n191 = property on="Image" class="IntGraph (strict)"("Active Cursor"=u32 1, "Cursor.Visible"=w391) -> ()  [unwired: 2 in, 2 out]
                              n192 = local write "Bin (n x n)"(w387) -> ()
                            }
                          }
                          n193 = local read "Previous Bin"() -> (w355:u16)
                        }
                        frame #2 {
                          n194 = local read "x pixels"() -> (w409:i32)
                          n195 = local read "Bin (n x n)"() -> (w410:u16)
                          n196 = call "subUpdateCameraBin_NW348.vi"("Bin (n x n)"=w401, "Previous bin"=w400, "Error in (no error)"=w426, "ROI in"=w424, "Handle in"=w425) -> ("Error out"=w422:errorcluster, "ROI out"=w395:T1, "Handle out"=w423:u32)  [unwired: 2 in, 2 out]
                          n197 = local read "Bin (n x n)"() -> (w398:u16)
                          n198 = local read "x pixels"() -> (w397:i32)
                          n199 = local read "Bin (n x n)"() -> (w394:u16)
                          n200 = call "subImageROI2CameraROI_NW348.vi"("image ROI"=w395) -> ("camera ROI"=w421:T1)
                          n201 = Unbundle By Name(w395) -> ("x offset"=w413:i32, "y offset"=w414:i32, "x width"=w416:i32, "y width"=w415:i32)
                          n202 = local write "ROI"(w395) -> ()
                          n203 = Divide(x=w409, y=w410) -> (x/y=w408:dbl)
                          n204 = call "subUpdateLocIndicator_NW348.vi"("ROI"=w395, "pixel range"=w408) -> ("Graph scale"=w407:T8, "Location indicator"=w402:u16[][])  [unwired: 8 in]
                          n205 = Divide(x=w397, y=w398) -> (x/y=w396:dbl)
                          n206 = Unbundle By Name(w407) -> ("X min"=w406:dbl, "Y min"=w405:dbl, "X max"=w404:dbl, "Y max"=w403:dbl)
                          n207 = call <userlib>:"tm_setarea.vi"("error in (no error)"=w422, "Sub Region"=w421, "Handle in"=w423) -> ("error out"=w419:errorcluster, "Handle out"=w420:u32)  [unwired: 7 in]
                          n208 = local write "Location indicator"(w402) -> ()
                          n209 = Add(x=w416, y=w413) -> (x+y=w412:i32)
                          n210 = call "subGetMaxCameraRate_cokeCan.vi"("Bin (n x n)"=w394, "ROI"=w395, "Binned pixels"=w396) -> ("max frame rate (Hz)"=→"max frame rate (Hz)":dbl)  [unwired: 8 in]
                          n211 = Add(x=w415, y=w414) -> (x+y=w411:i32)
                          n212 = property on="Image" class="IntGraph (strict)"("XScale.Minimum"=w406, "YScale.Minimum"=w405, "XScale.Maximum"=w404, "YScale.Maximum"=w403) -> ()  [unwired: 2 in, 2 out]
                          n213 = property on="Image" class="IntGraph (strict)"("Active Cursor"=u32 0, "Cursor.Cursor X"=w413, "Cursor.Cursor Y"=w414) -> ()  [unwired: 2 in, 2 out]
                          n214 = property on="Image" class="IntGraph (strict)"("Active Cursor"=u32 1, "Cursor.Cursor X"=w412, "Cursor.Cursor Y"=w411) -> ()  [unwired: 2 in, 2 out]
                        }
                      }
                      n215 = call <userlib>:"tm_preparecapture.vi"("error in (no error)"=w331, "Capture mode"=w338, "Handle in"=w332) -> ("error out"=w337:errorcluster, "Buffer"=w333:T4, "Handle out"=w336:u32)  [unwired: 5 in, 1 out]
                      n216 = call <userlib>:"tm_startcapture_b.vi"("error in (no error)"=w337, "Handle in"=w336) -> ("error out"=w334:errorcluster, "Handle out"=w335:u32)  [unwired: 8 in]
                    }
                    event "Define ROI": Value Change {
                      n217 = event-data() -> ()  [unwired: 1 in, 1 out]
                      n218 = case shown="True" "Define ROI" {
                        frame False {
                          w431 = FALSE ("Cursor.Visible")
                          n219 = property on="Image" class="IntGraph (strict)"("Active Cursor"=u32 0, "Cursor.Visible"=w431) -> ()  [unwired: 2 in, 2 out]
                          n220 = property on="Image" class="IntGraph (strict)"("Active Cursor"=u32 1, "Cursor.Visible"=w431) -> ()  [unwired: 2 in, 2 out]
                        }
                        frame True {
                          w434 = TRUE ("Cursor.Visible")
                          n221 = property on="Image" class="IntGraph (strict)"() -> ("XScale.Minimum"=w436:dbl, "YScale.Minimum"=w435:dbl, "XScale.Maximum"=w438:dbl, "YScale.Maximum"=w437:dbl)  [unwired: 2 in, 2 out]
                          n222 = property on="Image" class="IntGraph (strict)"("Active Cursor"=u32 0, "Cursor.Visible"=w434, "Cursor.Cursor X"=w436, "Cursor.Cursor Y"=w435) -> ()  [unwired: 2 in, 2 out]
                          n223 = property on="Image" class="IntGraph (strict)"("Active Cursor"=u32 1, "Cursor.Visible"=w434, "Cursor.Cursor X"=w438, "Cursor.Cursor Y"=w437) -> ()  [unwired: 2 in, 2 out]
                        }
                      }
                    }
                    event "Previous ROI 2": Value Change {
                      w441 = FALSE ("Define ROI")
                      w455 = 1 items=["Snap", "Sequence"] ("Capture mode")
                      w470 = 1 items=["BINNING"=1, "BITS PER CHANNEL"=2, "ACTIVE VIEW INDEX"=3, "CCD MODE"=4, "SENSOR MODE"=5, "READOUT MODE"=6, "EXPOSURE TIME"=7, "CONTRAST GAIN"=8, "CONTRAST OFFSET"=9, "LIGHT MODE"=10, "SENSITIVITY"=11, "WHITE BALANCE"=12, "PHOTON IMAGING MODE"=13, "HIGH DYNAMIC RANGE MODE"=14, "TRIGGER SOURCE"=15, "TRIGGER ACTIVE"=16, "TRIGGER MODE"=17, "TRIGGER POLARITY"=18, "TRIGGER GLOBAL EXPOSURE"=19, "FIRST TRIGGER BEHAVIOR"=20, "TRIGGER TIMES"=21, "OUTPUT TRIGGER POLARITY"=22, "OUTPUT TRIGGER DELAY"=23, "OUTPUT TRIGGER PERIOD"=24, "TEMPERATURE"=25, "TEMPERATURE TARGET"=26, "SENSOR COOLER FAN"=27, "MECHANICAL SHUTTER"=28, "BACK FOCUS POSITION"=29, "FRAMEBUNDLE MODE"=30, "FRAMEBUNDLE NUMBER"=31, "LINEBUNDLE HEIGHT"=32, "TRIGGER CONNECTOR"=33, "IMAGE PIXEL TYPE"=34] ("Parameter")
                      w471 = u16 2 items=["Full ROI", "Central quad", "Custom ROI"] ("ROI selection")
                      n224 = event-data() -> ()  [unwired: 1 in, 1 out]
                      n225 = call <userlib>:"tm_stopcapture.vi"("error in (no error)"=w443, "Handle in"=w444) -> ("error out"=w448:errorcluster, "Handle out"=w447:u32)  [unwired: 8 in]
                      n226 = local write "Define ROI"(w441) -> ()
                      n227 = local write "Previous ROI 2"(w441) -> ()
                      n228 = property on="Image" class="IntGraph (strict)"("Active Cursor"=u32 0, "Cursor.Visible"=w441) -> ()  [unwired: 2 in, 2 out]
                      n229 = property on="Image" class="IntGraph (strict)"("Active Cursor"=u32 1, "Cursor.Visible"=w441) -> ()  [unwired: 2 in, 2 out]
                      n230 = call <userlib>:"tm_unpreparecapture.vi"("error in (no error)"=w448, "Handle in"=w447) -> ("error out"=w445:errorcluster, "Handle out"=w446:u32)  [unwired: 8 in]
                      n231 = stacked-sequence {
                        seq-local: [w475 _ _] -> [_ _ w479]
                        seq-local: [w474 _ _] -> [_ _ w478]
                        tunnel: [_ w477 _] -> w467
                        tunnel: [_ w476 _] -> w459
                        frame #0 {
                          n232 = local read "ROI"() -> (w475:T1)
                          n233 = local read "Bin (n x n)"() -> (w474:u16)
                        }
                        frame #1 {
                          n234 = local read "Previous ROI"() -> (w476:T1)
                          n235 = local read "Previous Bin"() -> (w477:u16)
                          n236 = local write "Bin (n x n)"(w477) -> ()
                          n237 = local write "ROI"(w476) -> ()
                        }
                        frame #2 {
                          n238 = local write "Previous ROI"(w479) -> ()
                          n239 = local write "Previous Bin"(w478) -> ()
                        }
                      }
                      n240 = local write "ROI selection"(w471) -> ()
                      n241 = call <userlib>:"tm_setparameter.vi"("error in (no error)"=w445, "Value in"=w467, "Parameter"=w470, "Handle in"=w446) -> ("error out"=w457:errorcluster, "Handle out"=w456:u32)  [unwired: 6 in]
                      n242 = local read "x pixels"() -> (w468:i32)
                      n243 = Divide(x=w468, y=w467) -> (x/y=w469:dbl)
                      n244 = call "subImageROI2CameraROI_NW348.vi"("image ROI"=w459) -> ("camera ROI"=w458:T1)
                      n245 = call "subUpdateLocIndicator_NW348.vi"("ROI"=w459, "pixel range"=w469) -> ("Graph scale"=w465:T8, "Location indicator"=w466:u16[][])  [unwired: 8 in]
                      n246 = call <userlib>:"tm_setarea.vi"("error in (no error)"=w457, "Sub Region"=w458, "Handle in"=w456) -> ("error out"=w451:errorcluster, "Handle out"=w452:u32)  [unwired: 7 in]
                      n247 = local write "Location indicator"(w466) -> ()
                      n248 = Unbundle By Name(w465) -> ("X min"=w464:dbl, "Y min"=w463:dbl, "X max"=w462:dbl, "Y max"=w461:dbl)
                      n249 = call <userlib>:"tm_preparecapture.vi"("error in (no error)"=w451, "Capture mode"=w455, "Handle in"=w452) -> ("error out"=w453:errorcluster, "Buffer"=w442:T4, "Handle out"=w454:u32)  [unwired: 5 in, 1 out]
                      n250 = property on="Image" class="IntGraph (strict)"("XScale.Minimum"=w464, "YScale.Minimum"=w463, "XScale.Maximum"=w462, "YScale.Maximum"=w461) -> ()  [unwired: 2 in, 2 out]
                      n251 = Wait (ms)(milliseconds to wait=u32 200) -> ()  [unwired: 1 out]
                      n252 = call <userlib>:"tm_startcapture_b.vi"("error in (no error)"=w453, "Handle in"=w454) -> ("error out"=w449:errorcluster, "Handle out"=w450:u32)  [unwired: 8 in]
                    }
                    event "# frames": Value Change {
                      n253 = event-data() -> ()  [unwired: 1 in, 1 out]
                      n254 = local read "Exposure (msec)"() -> (w484:T3)
                      n255 = local read "# frames"() -> (w485:u32)
                      n256 = Multiply(x=w485, y=w484) -> (x*y=w483:T3)
                      n257 = Divide(x=w483, y=1000) -> (x/y=→"Total time (sec)":T3)
                    }
                  }
                  n258 = local read "Enter Live Mode"() -> (w79:bool)
                  n259 = Wait (ms)(milliseconds to wait=u32 50) -> ()  [unwired: 1 out]
                }
                n260 = call <userlib>:"tm_stopcapture.vi"("error in (no error)"=w60, "Handle in"=w59) -> ("error out"=w61:errorcluster, "Handle out"=w62:u32)  [unwired: 8 in]
                n261 = call <userlib>:"tm_unpreparecapture.vi"("error in (no error)"=w61, "Handle in"=w62) -> ("error out"=w58:errorcluster)  [unwired: 8 in, 1 out]
                n262 = local write "Camera Error"(w58) -> ()
              }
            }
          }
          frame #1 {
            # "Snap and Save Frame"
          }
          frame #2 {
            # "Record Video Frame"
          }
        }
      }
    }
    frame #2 {
      n263 = local read "Camera Error"() -> (w487:errorcluster)
      n264 = call <userlib>:"tm_closecamera.vi"("error in (no error)"=w487, "Handle in"=u32 0) -> ("error out"=w489:errorcluster)  [unwired: 9 in]
      n265 = call <userlib>:"tm_deinitialize.vi"("error in (no error)"=w489) -> ("error out"=w486:errorcluster)  [unwired: 10 in]
      n266 = local write "Camera Error"(w486) -> ()
    }
  }
